vi "Error_calc.vi"(9 "Error Type":enum16{"MSE", "MAE"}(ring)=enum."MAE", 10 "Target":dbl, 11 "Data":dbl) -> (3 "Error":dbl)   [LabVIEW 2018]
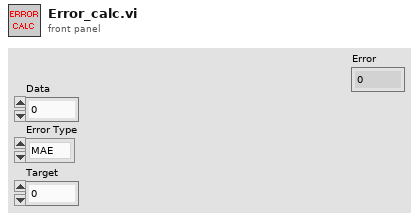
[diagram p1: front panel]
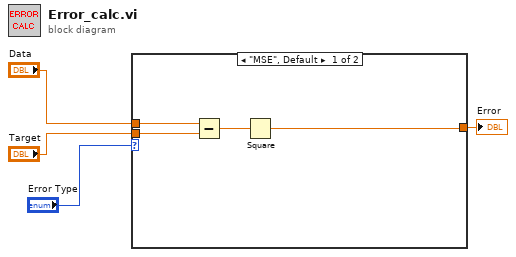
[diagram p0: block diagram]
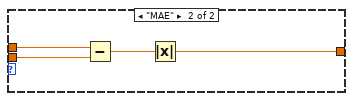
[diagram p2: hidden frame]
diagram:
  n1 = case shown="\"MSE\", Default" "Error Type" {
    tunnel: "Data" -> [w8 w12]
    tunnel: "Target" -> [w7 w11]
    tunnel: [w5 w9] -> w1
    frame "MSE", Default {
      n2 = Subtract(x=w8, y=w7) -> (x-y=w6:dbl)
      n3 = Square(x=w6) -> (x^2=w5:dbl)
    }
    frame "MAE" {
      n4 = Subtract(x=w12, y=w11) -> (x-y=w10:dbl)
      n5 = Absolute Value(x=w10) -> (abs(x)=w9:dbl)
    }
  }
  "Error" <- w1
